vi "Parse CSV (Polymorphic) (Mark Siekmeier's conflicted copy 2013-04-30).vi"   [LabVIEW 2012]
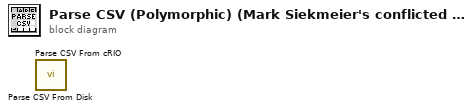
[diagram p0: block diagram]
diagram:
  n1 = call "Parse CSV From Disk.vi"() -> ()  [unwired: 5 in, 1 out]
  n2 = call "Parse CSV From cRIO.vi"() -> ()  [unwired: 5 in, 1 out]
